vi "SimulatedHallPulse.vi"(4 "AO Rate":dbl=100000.0, 5 "Buffer Size":i32=100000, 6 "error in (no error)":errorcluster, 7 "RPM":dbl=0.1, 9 "Pulse Params":T1={"Amplitude"=5.0, "Duty Cycle"=0.1, "Shape"=enum."Square"}) -> (0 "error out":errorcluster, 1 "RPM out":dbl=0.1, 3 "Waveform Graph":waveform(dbl)(graph))   [LabVIEW 2014]
uses:
  <vilib>/Analysis/1siggen.llb/Ramp Pattern by Samples.vi
  <vilib>/Waveform/WDTOps.llb/WDT Append Waveforms DBL.vi
  <vilib>/Analysis/NI_AALBase.lvlib
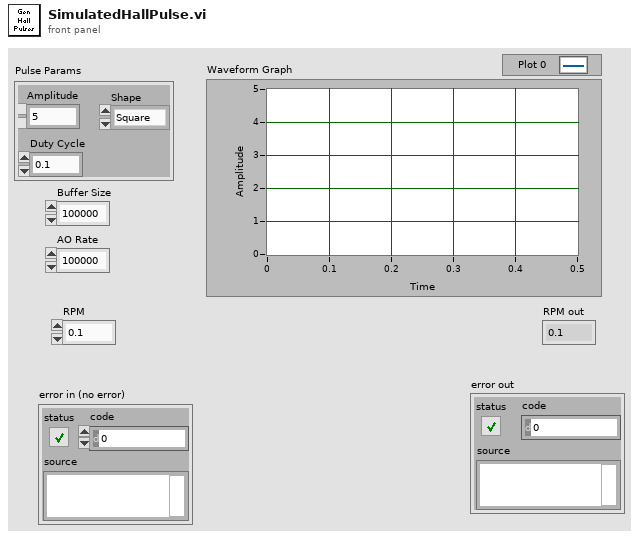
[diagram p1: front panel]
types:
  T1 = cluster{"Amplitude":dbl, "Duty Cycle":dbl, "Shape":enum16{"Square", "Cosine"}}
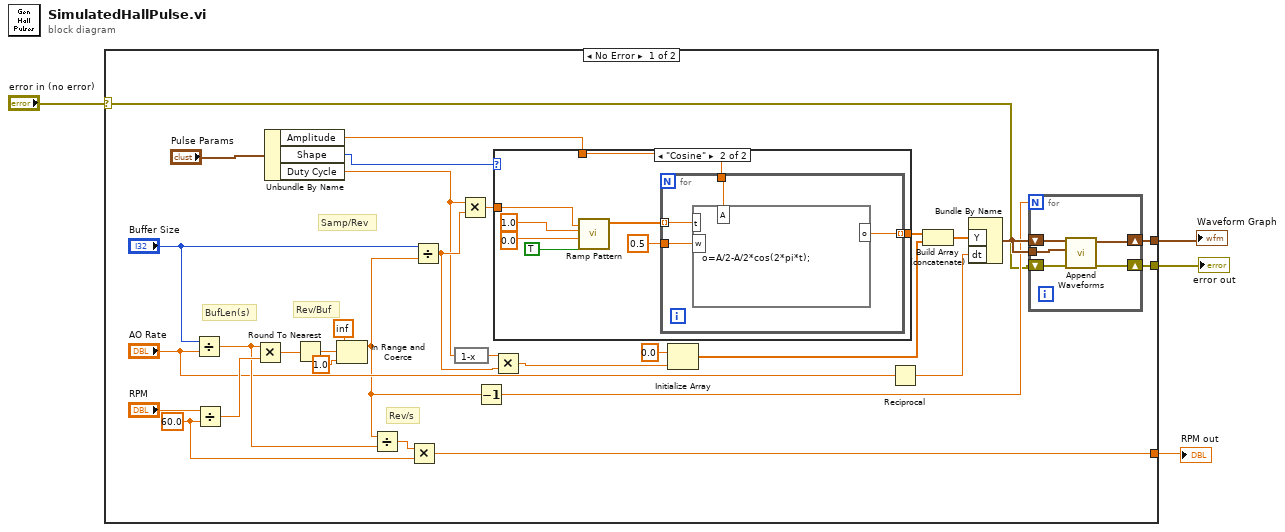
[diagram p0: block diagram]
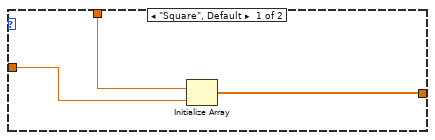
[diagram p2: hidden frame]
diagram:
  n1 = case shown="No Error" "error in (no error)" {
    selector: "error in (no error)" -> [w14 w56]
    tunnel: [w16 _] -> w4
    tunnel: [w15 w56] -> w2
    tunnel: [w13 _] -> w1
    frame No Error {
      w32 = 60.0 ("y")
      # "Samp/Rev"
      # "Rev/s"
      # "Rev/Buf"
      # "BufLen(s)"
      n2 = Divide(x="Buffer Size", y="AO Rate") -> (x/y=w31:dbl)
      n3 = Divide(x="RPM", y=w32) -> (x/y=w33:dbl)
      n4 = Multiply(x=w31, y=w33) -> (x*y=w34:dbl)
      n5 = Unbundle By Name("Pulse Params") -> ("Amplitude"=w8:dbl, "Shape"=w6:enum16{"Square", "Cosine"}, "Duty Cycle"=w7:dbl)
      n6 = Round To Nearest(number=w34) -> (nearest integer value=w12:dbl)
      n7 = In Range and Coerce(upper limit=inf, x=w12, lower limit=1.0) -> (coerced(x)=w10:dbl)  [unwired: 1 out]
      n8 = Divide(x=w10, y=w31) -> (x/y=w30:dbl)
      n9 = Multiply(x=w30, y=w32) -> (x*y=w13:dbl)
      n10 = Divide(x="Buffer Size", y=w10) -> (x/y=w26:dbl)
      n11 = expression code="1-x"(w7) -> (w27:dbl)
      n12 = Multiply(x=w7, y=w26) -> (x*y=w28:dbl)
      n13 = Decrement(x=w10) -> (x-1=w17:dbl)
      n14 = Multiply(x=w27, y=w26) -> (x*y=w25:dbl)
      n15 = case shown="\"Cosine\"" w6 {
        tunnel: w28 -> [w37 w41]
        tunnel: [w38 w40] -> w23
        tunnel: w8 -> [w36 w39]
        frame "Square", Default {
          n16 = Initialize Array(w36, w37) -> (w38:dbl[])
        }
        frame "Cosine" {
          n17 = call-poly <vilib>:"Ramp Pattern.vi"("exclude end?"=TRUE, "start"=0.0, "end"=1.0, "samples"=w41) -> ("Ramp Pattern"=w42:dbl[])  [unwired: 6 in, 1 out]
          n18 = for {
            tunnel: w42 -> [w50] mode=indexing
            tunnel: 0.5 ("input variable") -> [w49]
            tunnel: w39 -> [w48]
            tunnel: [w47] -> w40 mode=indexing
            n19 = formula code="o=A/2-A/2*cos(2*pi*t);"("t"=w50, "w"=w49, "A"=w48) -> ("o"=w47:dbl)
          }
        }
      }
      n20 = Initialize Array(0.0 ("element"), w25) -> (w22:dbl[])
      n21 = Reciprocal(x="AO Rate") -> (1/x=w19:dbl)
      n22 = Build Array (concatenate)(w23, w22) -> (w21:dbl[])
      n23 = Bundle By Name("Y"=w21, "dt"=w19) -> (w18:waveform(dbl))  [unwired: 1 in]
      n24 = for {
        N: w17 -> [_]
        shift-right: [w54] -> w16
        shift-left: w18 -> [w55]
        tunnel: w18 -> [w53]
        shift-right: [w52] -> w15
        shift-left: w14 -> [w51]
        n25 = call-poly <vilib>:"Append Waveforms.vi"("error in (no error)"=w51, "waveform B"=w53, "waveform A"=w55) -> ("error out"=w52:errorcluster, "waveform out"=w54:waveform(dbl))  [unwired: 7 in]
      }
    }
    frame Error {
    }
  }
  "Waveform Graph" <- w4
  "error out" <- w2
  "RPM out" <- w1
